vi "_attribute_write_int64.vi"(5 "Repeated Capability":string, 7 "Attribute":T1={"Identifier"="", "Descriptive Name"="", "Data Type"=enum."Integer 32", "Command"="", "Access"=enum."Read/Write", "Range Table"="", "Read Callback"="", "Write Callback"="", "Supported Models"="", "Instrument Options"="", "Index"=0, "OPC Wait"=FALSE, "No Status Check"=FALSE, "Cache Only"=FALSE}, 8 "error in":errorcluster caption="error in (no error)", 10 "Int64 in":i64, 11 "VISA resource name":refnum<visa-resource-name>) -> (0 "error out":errorcluster, 3 "VISA resource name out":refnum<visa-resource-name>)   [LabVIEW 2020, in "Rohde&Schwarz RTx Oscilloscopes.lvlib" / "rsidr_core.lvlib"]
uses:
  rsidr_core.lvlib
  type_Attribute.ctl
  type_Attribute_Data_Type.ctl
  type_ReadWriteAccess.ctl
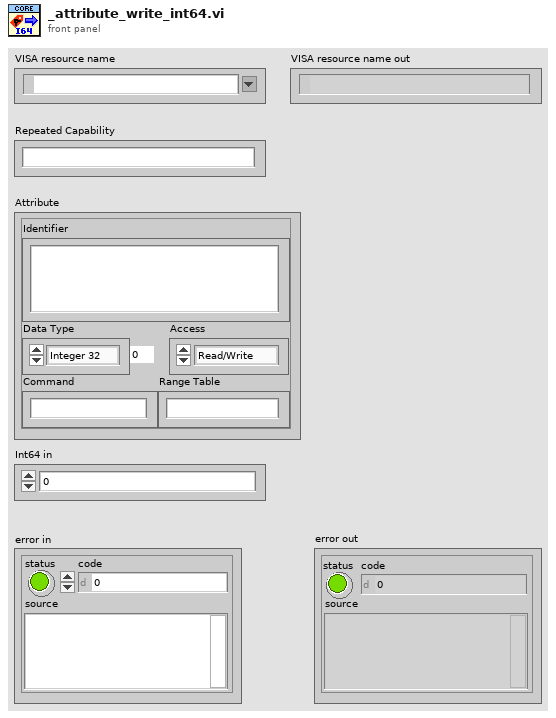
[diagram p1: front panel]
types:
  T1 = typedef "Rohde&Schwarz RTx Oscilloscopes.lvlib/rsidr_core.lvlib/type_Attribute.ctl" = cluster{"Identifier":string, "Descriptive Name":string, "Data Type":T2, "Command":string, "Access":T3, "Range Table":string, "Read Callback":string, "Write Callback":string, "Supported Models":string, "Instrument Options":string, "Index":i32, "OPC Wait":bool, "No Status Check":bool, "Cache Only":bool}
  T2 = typedef "Rohde&Schwarz RTx Oscilloscopes.lvlib/rsidr_core.lvlib/type_Attribute_Data_Type.ctl" = enum16{"Integer 32", "Double", "String", "Boolean", "None", "Integer 64", "RawString"}
  T3 = typedef "Rohde&Schwarz RTx Oscilloscopes.lvlib/rsidr_core.lvlib/type_ReadWriteAccess.ctl" = enum16{"Read Only", "Write Only", "Read/Write"}
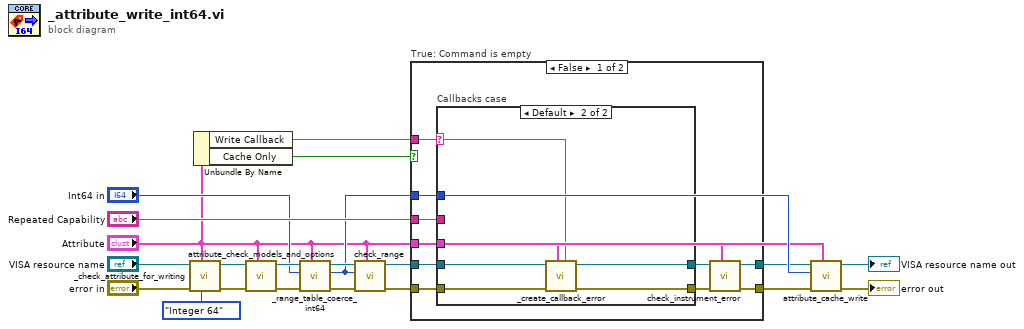
[diagram p0: block diagram]
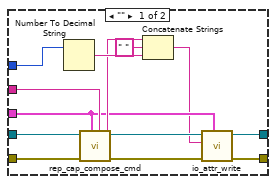
[diagram p2: hidden frame]
diagram:
  n1 = call "_check_attribute_for_writing.vi"("Expected Data Type"=type_Attribute_Data_Type."Integer 64" ("Data Type"), "Attribute"="Attribute", "error in"="error in", "VISA resource name"="VISA resource name") -> ("error out"=w12:errorcluster, "VISA resource name out"=w11:refnum<visa-resource-name>)  [unwired: 6 in]
  n2 = Unbundle By Name("Attribute") -> ("Write Callback"=w13:string, "Cache Only"=w1:bool)
  n3 = call "attribute_check_models_and_options.vi"("Attribute"="Attribute", "error in"=w12, "VISA resource name"=w11) -> ("error out"=w10:errorcluster, "VISA resource name out"=w9:refnum<visa-resource-name>)  [unwired: 6 in, 1 out]
  n4 = call "_range_table_coerce_int64.vi"("Attribute"="Attribute", "error in"=w10, "Int64 in"="Int64 in", "VISA resource name"=w9) -> ("error out"=w8:errorcluster, "Int64 out"=w5:i64, "VISA resource name out"=w7:refnum<visa-resource-name>)  [unwired: 5 in]
  n5 = call "check_range.vi"("Attribute"="Attribute", "error in"=w8, "Value to check"=w5, "VISA resource name"=w7) -> ("error out"=w16:errorcluster, "VISA resource name out"=w15:refnum<visa-resource-name>)  [unwired: 6 in]
  n6 = case "True: Command is empty" shown="False" w1 {
    tunnel: "Repeated Capability" -> [w31 _]
    tunnel: w16 -> [w30 w51]
    tunnel: w15 -> [w29 w52]
    tunnel: w5 -> [w28 _]
    tunnel: "Attribute" -> [w22 _]
    tunnel: [w23 w52] -> w2
    tunnel: [w24 w51] -> w3
    tunnel: w13 -> [w27 _]
    frame False {
      n7 = case "Callbacks case" shown="Default" w27 {
        selector: w27 -> [_ w45]
        tunnel: w28 -> [w37 _]
        tunnel: w29 -> [w43 w49]
        tunnel: w30 -> [w41 w50]
        tunnel: w31 -> [w38 _]
        tunnel: [w40 w47] -> w25
        tunnel: [w39 w48] -> w26
        tunnel: w22 -> [w33 w46]
        frame "" {
          n8 = Number To Decimal String(number=w37) -> (decimal integer string=w35:string)  [unwired: 1 in]
          n9 = call "rep_cap_compose_cmd.vi"("Repeated Capability"=w38, "Attribute"=w33, "error in"=w41, "VISA resource name"=w43) -> ("error out"=w42:errorcluster, "Command out"=w34:string, "VISA resource name out"=w44:refnum<visa-resource-name>)  [unwired: 5 in]
          n10 = Concatenate Strings(w34, " ", w35) -> (w32:string)
          n11 = call "io_attr_write.vi"("Attribute"=w33, "error in"=w42, "write buffer"=w32, "VISA resource name"=w44) -> ("error out"=w39:errorcluster, "VISA resource name out"=w40:refnum<visa-resource-name>)  [unwired: 6 in]
        }
        frame Default {
          n12 = call "_create_callback_error.vi"("Callback Name"=w45, "Attribute"=w46, "error in"=w50, "VISA resource name"=w49) -> ("error out"=w48:errorcluster, "VISA resource name out"=w47:refnum<visa-resource-name>)  [unwired: 6 in]
        }
      }
      n13 = call "check_instrument_error.vi"("Attribute"=w22, "error in"=w26, "VISA resource name"=w25) -> ("error out"=w24:errorcluster, "VISA resource name out"=w23:refnum<visa-resource-name>)  [unwired: 7 in]
    }
    frame True {
    }
  }
  n14 = call "attribute_cache_write.vi"("Attribute"="Attribute", "error in"=w3, "Value in"=w5, "VISA resource name"=w2) -> ("error out"=→"error out":errorcluster, "VISA resource name out"=→"VISA resource name out":refnum<visa-resource-name>)  [unwired: 6 in]
